vi "Acquisition Message Loop.vi"(8 "error in (no error)":errorcluster, 9 "queue out":refnum<queue>, 10 "Data Notifier":refnum<notifier>, 11 "Message Queues":T1) -> (0 "error out":errorcluster)   [LabVIEW 2022 SP3, in "Acquisition.lvlib"]
doc: "Message loop for handling messages pertaining to the acquisition of data from the hardware."
uses:
  Acquisition.lvlib
  support/Message Queue/Message Cluster.ctl
  Acquisition State.ctl
  GlobalVariable/GlobalDisconnected.vi
  GlobalVariable/GlobalFirstRep.vi
  GlobalVariable/GlobalPowerByTime.vi
  GlobalVariable/GlobalPosXbyTime.vi
  GlobalVariable/GlobalPosYbyTime.vi
  GlobalVariable/GlobalProfileByTime.vi
  GlobalVariable/Globalt0.vi
  support/Message Queue/Enqueue Message (Single).vi
  GlobalVariable/GlobalLongueurOnde.vi
  GlobalVariable/GlobalTimeStep.vi
  <vilib>/Utility/error.llb/Error Cluster From Error Code.vi
  <vilib>/ErrorRing/Error Ring.xnode
  support/Message Queue/Message Queue.lvlib
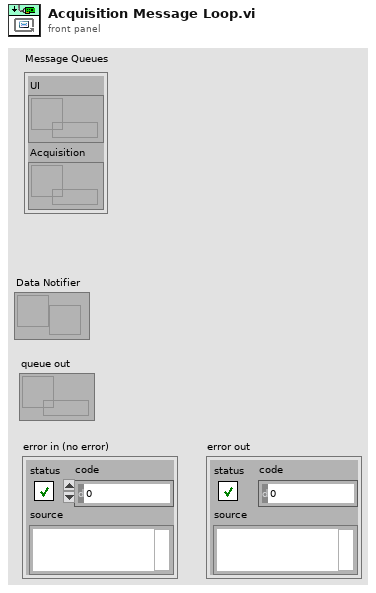
[diagram p1: front panel]
types:
  T1 = cluster{"UI":refnum<queue>, "Acquisition":refnum<queue>}
  T2 = typedef "Acquisition.lvlib/Acquisition State.ctl" = enum16{"Idle", "Acquiring"}
  T3 = enum16{"open", "replace", "create", "open or create", "replace or create", "replace or create with confirmation"}
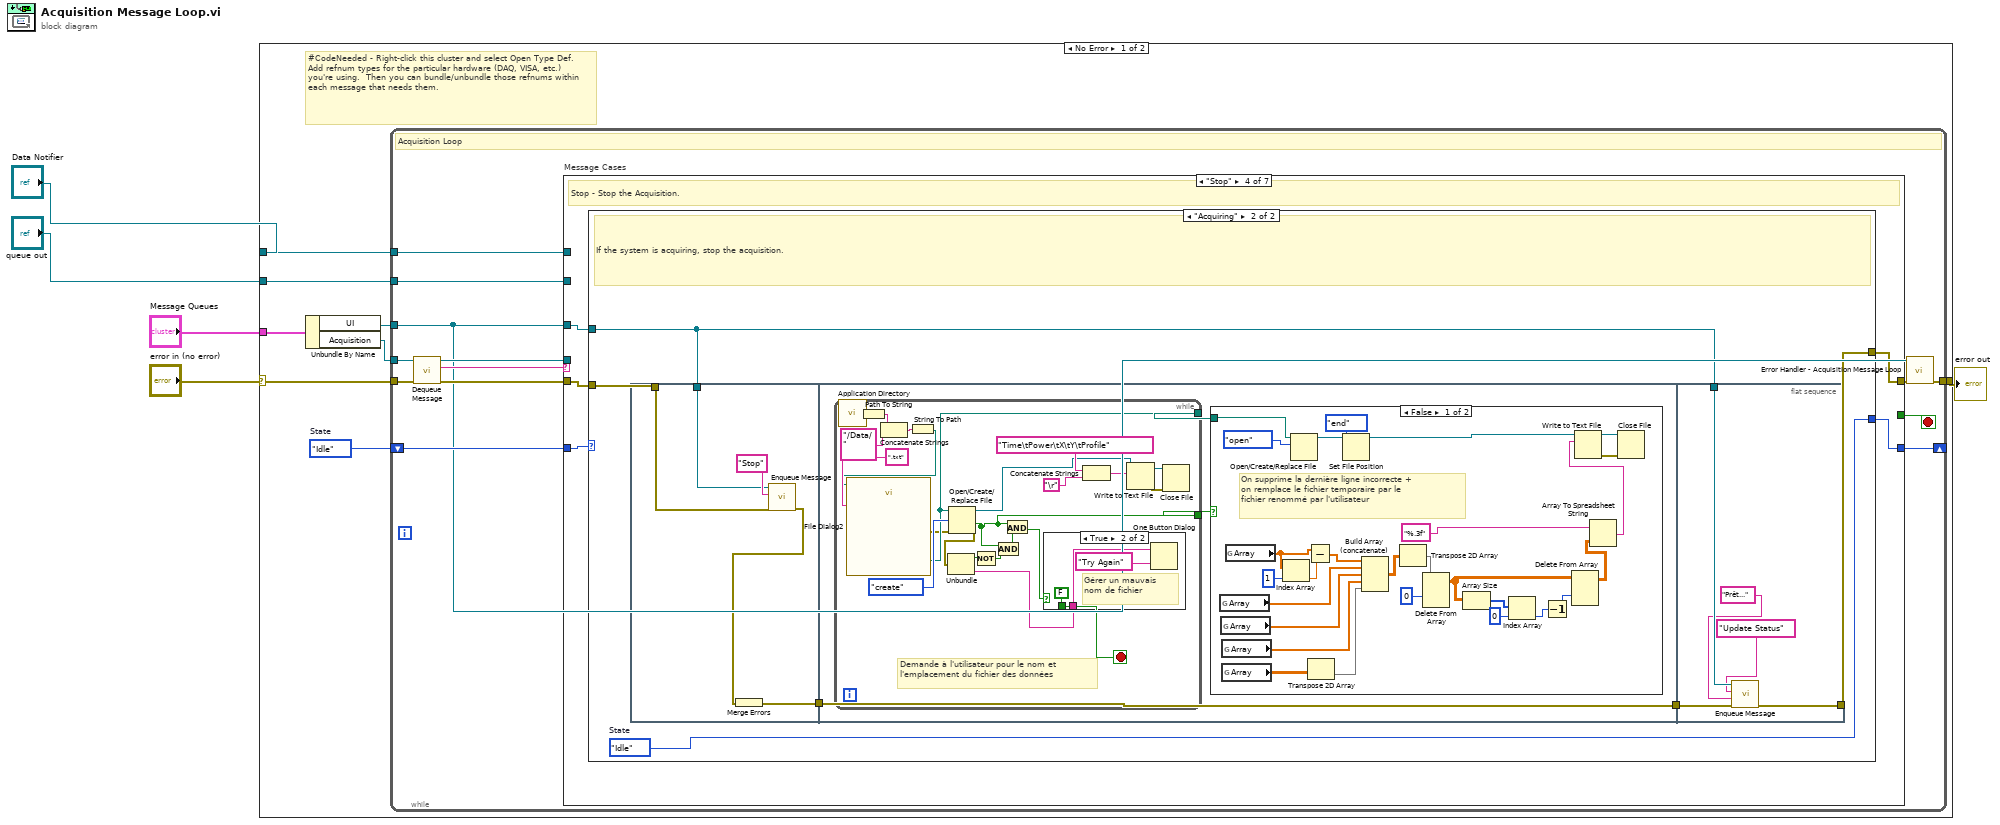
[diagram p0: block diagram]
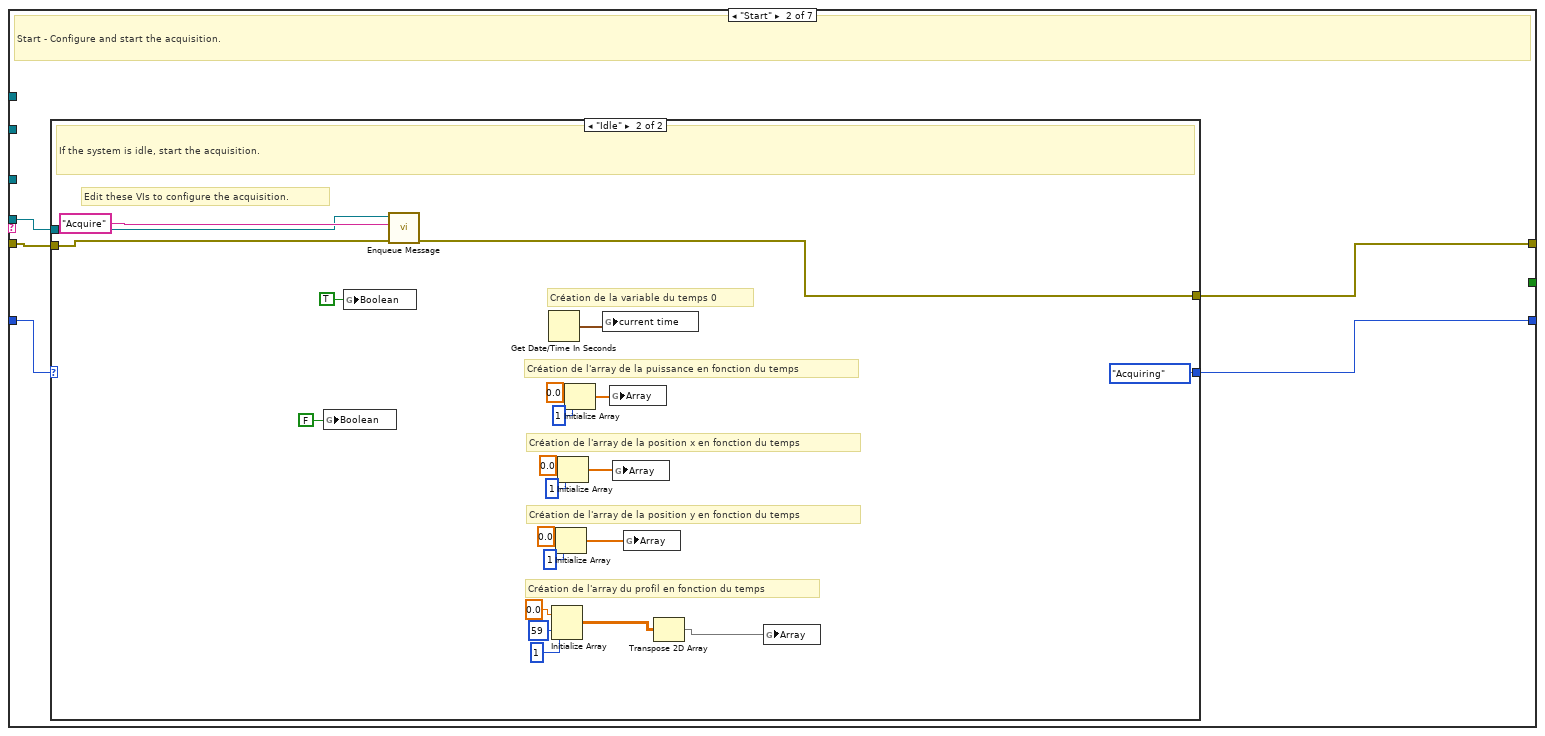
[diagram p3: hidden frame]
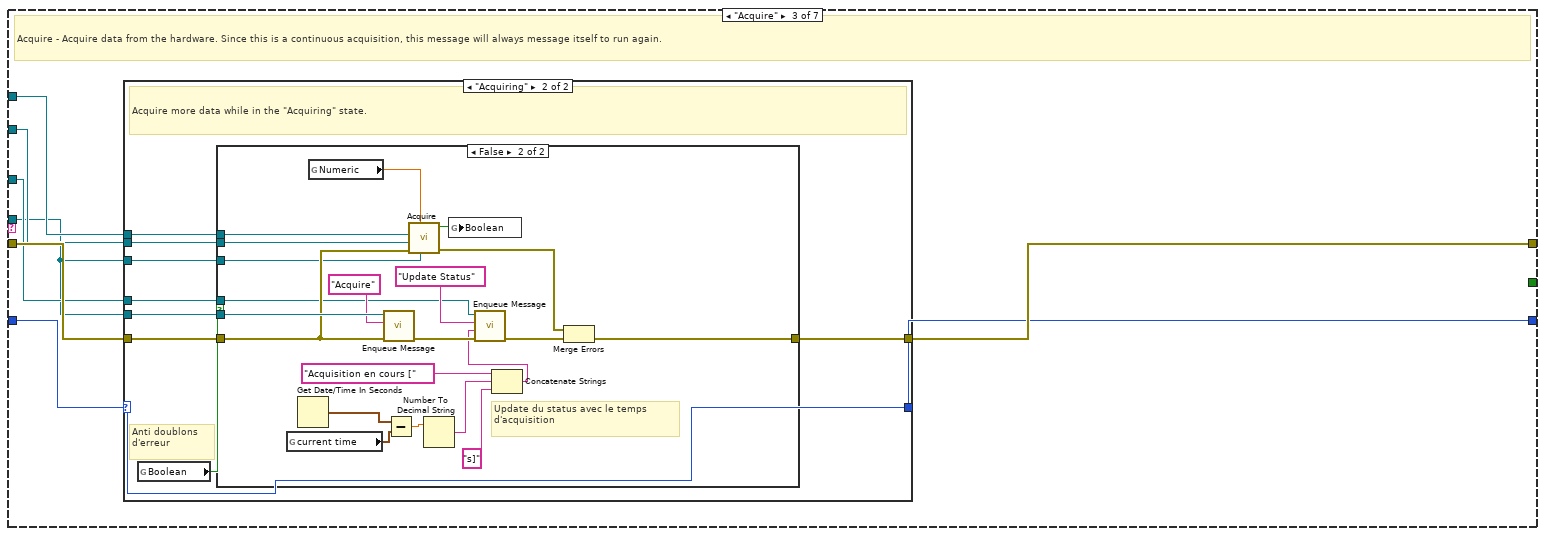
[diagram p5: hidden frame]
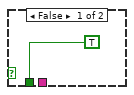
[diagram p10: hidden frame]
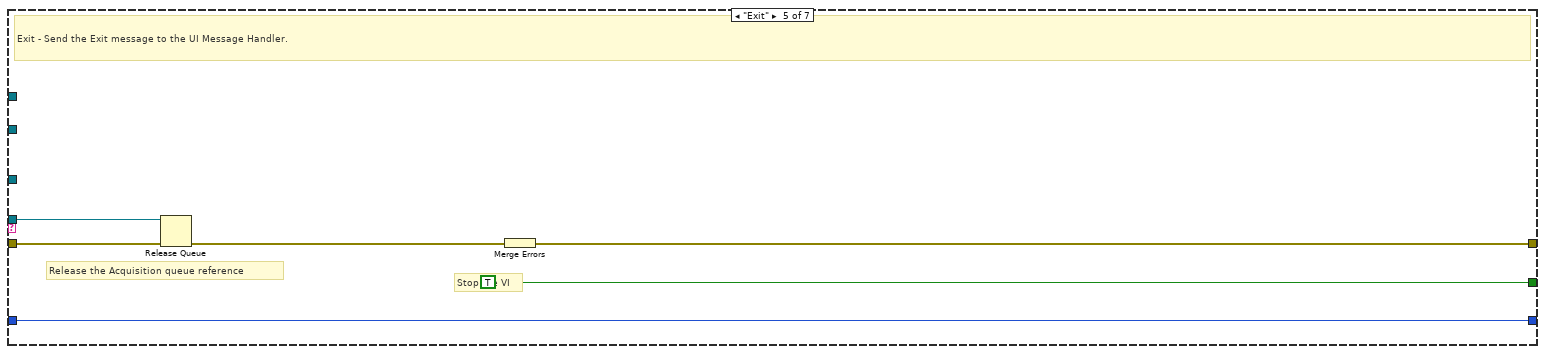
[diagram p11: hidden frame]
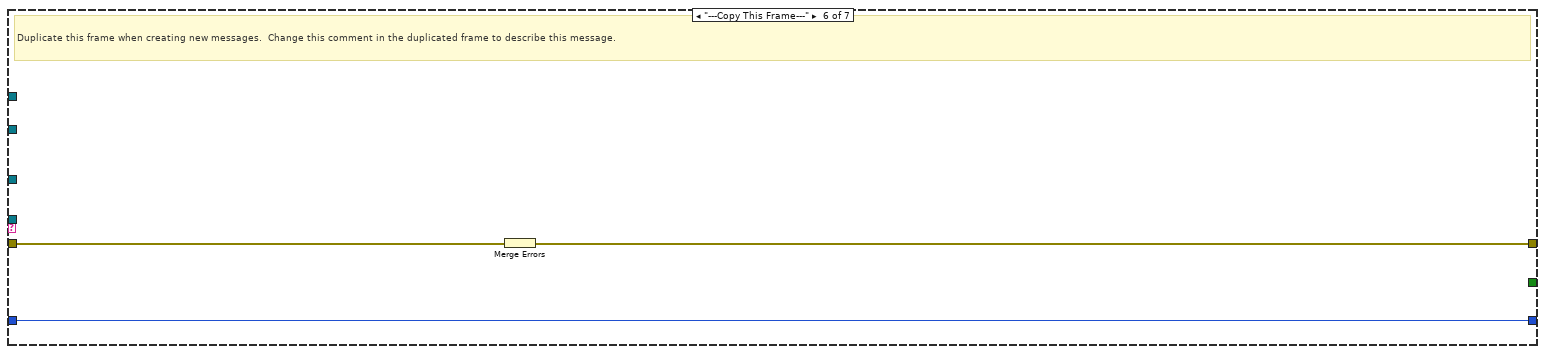
[diagram p12: hidden frame]
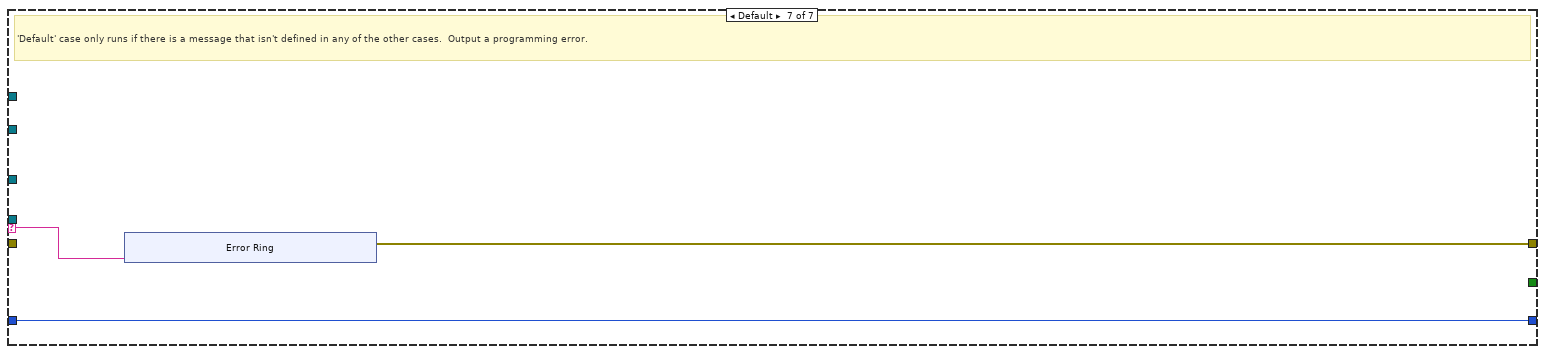
[diagram p13: hidden frame]
diagram:
  n1 = case shown="No Error" "error in (no error)" {
    selector: "error in (no error)" -> [w10 w198]
    tunnel: "Message Queues" -> [w13 _]
    tunnel: [w11 w198] -> w4
    tunnel: "Data Notifier" -> [w8 _]
    tunnel: "queue out" -> [w7 _]
    frame No Error {
      w6 = Acquisition_State."Idle"  # State
      # "#CodeNeeded - Right-click this cluster and select Open Type Def.  Add refnum types for the particular hardware (DAQ, VISA, etc.) you're using.  Then you can bundle/unbundle those refnums within each message that needs them."
      n2 = Unbundle By Name(w13) -> ("UI"=w9:refnum<queue>, "Acquisition"=w12:refnum<queue>)
      n3 = while {
        tunnel: w12 -> [w14]
        tunnel: w9 -> [w15]
        tunnel: w8 -> [w22]
        tunnel: w7 -> [w21]
        shift-right: [w19] -> _
        shift-left: w6 -> [w20]
        tunnel: w10 -> [w25]
        tunnel: [w18] -> w11
        stop <- w26 stop-if-true
        # "Acquisition Loop"
        n4 = call "Dequeue Message.vi"("error in (no error)"=w25, "Message Queue"=w14) -> ("error out"=w24:errorcluster, "Message"=w23:string, "dup Message Queue"=w16:refnum<queue>)  [unwired: 6 in, 1 out]
        n5 = case "Message Cases" shown="\"Stop\"" w23 {
          selector: w23 -> [_ _ _ _ _ _ w188]
          tunnel: w16 -> [_ w31 w58 _ w180 _ _]
          tunnel: w24 -> [w28 w32 w64 w102 w182 w187 _]
          tunnel: [w28 w33 w65 w100 w183 w186 w189] -> w17
          tunnel: [_ _ _ _ TRUE _ _] -> w26
          tunnel: w15 -> [_ _ w59 w101 _ _ _]
          tunnel: w22 -> [_ _ w63 _ _ _ _]
          tunnel: w21 -> [_ _ w62 _ _ _ _]
          tunnel: w20 -> [w27 w29 w60 w103 w179 w185 w190]
          tunnel: [w27 w30 w61 w99 w179 w185 w190] -> w19
          frame "Initialize" {
            # "Initialize  - Initialize is currently a no-op.  The hardware initialization takes place in the 'Start' message."
          }
          frame "Start" {
            # "Start - Configure and start the acquisition."
            n6 = case shown="\"Idle\"" w29 {
              selector: w29 -> [w34 _]
              tunnel: [w35 w53] -> w33
              tunnel: w32 -> [w35 w57]
              tunnel: w31 -> [_ w54]
              tunnel: [w34 Acquisition_State."Acquiring" ("Acquisition State")] -> w30
              frame "Acquiring" {
                # "The system is already acquiring. Ignore the \"Start\" message."
              }
              frame "Idle" {
                # "Création de la variable du temps 0"
                # "Création de l'array du profil en fonction du temps"
                # "Création de l'array de la position y en fonction du temps"
                # "Création de l'array de la position x en fonction du temps"
                # "Création de l'array de la puissance en fonction du temps"
                # "Edit these VIs to configure the acquisition."
                # "If the system is idle, start the acquisition."
                n7 = global write "GlobalDisconnected.vi" "Boolean"(FALSE) -> ()
                n8 = global write "GlobalFirstRep.vi" "Boolean"(TRUE ("Boolean")) -> ()
                n9 = call-poly "Enqueue Message.vi"("error in (no error)"=w57, "Message"="Acquire", "Message Queue"=w54) -> ("error out"=w53:errorcluster)  [unwired: 7 in, 1 out]
                n10 = Get Date/Time In Seconds() -> (seconds since 1Jan1904=w36:timestamp)
                n11 = Initialize Array(0.0, 59 ("dimension size"), 1 ("dimension size")) -> (w49:dbl[][])
                n12 = Initialize Array(0.0, 1) -> (w50:dbl[])
                n13 = Initialize Array(0.0, 1) -> (w51:dbl[])
                n14 = Initialize Array(0.0, 1) -> (w52:dbl[])
                n15 = global write "Globalt0.vi" "current time"(w36) -> ()
                n16 = global write "GlobalPowerByTime.vi" "Array"(w52) -> ()
                n17 = global write "GlobalPosXbyTime.vi" "Array"(w51) -> ()
                n18 = global write "GlobalPosYbyTime.vi" "Array"(w50) -> ()
                n19 = Transpose 2D Array(2D array=w49) -> (transposed array=w48:dbl[][])
                n20 = global write "GlobalProfileByTime.vi" "Array"(w48) -> ()
              }
            }
          }
          frame "Acquire" {
            # "Acquire - Acquire data from the hardware. Since this is a continuous acquisition, this message will always message itself to run again."
            n21 = case shown="\"Acquiring\"" w60 {
              selector: w60 -> [w66 w72]
              tunnel: [w67 w76] -> w65
              tunnel: w58 -> [_ w75]
              tunnel: w64 -> [w67 w71]
              tunnel: w63 -> [_ w74]
              tunnel: w62 -> [_ w73]
              tunnel: [w66 w72] -> w61
              tunnel: w59 -> [_ w70]
              tunnel: w58 -> [_ w69]
              frame "Idle" {
                # "Ignore \"Acquire\" messages when the acquisition is idle."
              }
              frame "Acquiring" {
                # "Anti doublons\nd'erreur"
                # "Acquire more data while in the \"Acquiring\" state."
                n22 = global read "GlobalDisconnected.vi" "Boolean"() -> (w68:bool)
                n23 = case shown="False" w68 {
                  tunnel: [w77 w98] -> w76
                  tunnel: w75 -> [_ w97]
                  tunnel: w74 -> [_ w94]
                  tunnel: w73 -> [_ w93]
                  tunnel: w71 -> [w77 w92]
                  tunnel: w70 -> [_ w81]
                  tunnel: w69 -> [_ w80]
                  frame True {
                  }
                  frame False {
                    # "Update du status avec le temps\nd'acquisition"
                    n24 = global read "Globalt0.vi" "current time"() -> (w87:timestamp)
                    n25 = Get Date/Time In Seconds() -> (seconds since 1Jan1904=w86:timestamp)
                    n26 = global read "GlobalLongueurOnde.vi" "Numeric"() -> (w79:dbl)
                    n27 = call-poly "Enqueue Message.vi"("error in (no error)"=w92, "Message"="Acquire", "Message Queue"=w97) -> ("error out"=w90:errorcluster)  [unwired: 7 in, 1 out]
                    n28 = Subtract(x=w86, y=w87) -> (x-y=w88:dbl)
                    n29 = call "Acquire.vi"("Acquisition"=w80, "Longueur d'onde"=w79, "error in (no error)"=w92, "Data Queue"=w93, "Data Notifier"=w94) -> ("error out"=w96:errorcluster, "Disconnected"=w78:bool)  [unwired: 5 in]
                    n30 = Number To Decimal String(number=w88) -> (decimal integer string=w85:string)  [unwired: 1 in]
                    n31 = global write "GlobalDisconnected.vi" "Boolean"(w78) -> ()
                    n32 = Concatenate Strings("Acquisition en cours [", w85, "s]" ("string")) -> (w83:string)
                    n33 = call-poly "Enqueue Message.vi"("error in (no error)"=w90, "Message Data"=w83, "Message"="Update Status", "Message Queue"=w81) -> ("error out"=w91:errorcluster)  [unwired: 6 in, 1 out]
                    n34 = Merge Errors(w96, w91) -> (w98:errorcluster)
                  }
                }
              }
            }
          }
          frame "Stop" {
            # "Stop - Stop the Acquisition."
            n35 = case shown="\"Acquiring\"" w103 {
              selector: w103 -> [w105 _]
              tunnel: w102 -> [w104 w110]
              tunnel: w101 -> [_ w106]
              tunnel: [w104 w109] -> w100
              tunnel: [w105 w108] -> w99
              frame "Idle" {
                # "The system is already idle. Ignore the \"Stop\" message."
              }
              frame "Acquiring" {
                w108 = Acquisition_State."Idle"  # State
                # "If the system is acquiring, stop the acquisition."
                n36 = flat-sequence {
                  tunnel: [w116] -> w111
                  tunnel: w106 -> [w113]
                  tunnel: w110 -> [w112]
                  tunnel: w111 -> [w118]
                  tunnel: [w118] -> w107
                  tunnel: [w177] -> w109
                  tunnel: w107 -> [w178]
                  tunnel: w106 -> [w176]
                  frame #0 {
                    n37 = call-poly "Enqueue Message.vi"("error in (no error)"=w112, "Message"="Stop", "Message Queue"=w113) -> ("error out"=w115:errorcluster)  [unwired: 7 in, 1 out]
                    n38 = Merge Errors(w115) -> (w116:errorcluster)
                  }
                  frame #1 {
                    n39 = while {
                      tunnel: [w164] -> w119
                      tunnel: [w154] -> w117
                      stop <- w160 stop-if-true
                      # "Demande à l'utilisateur pour le nom et\nl'emplacement du fichier des données"
                      n40 = call <vilib>:"Application Directory.vi"() -> ("Application Directory"=w167:path)
                      n41 = Path To String(path=w167) -> (string=w168:string)
                      n42 = Concatenate Strings(w168, "/Data/") -> (w169:string)
                      n43 = String To Path(string=w169) -> (path=w153:path)
                      n44 = call "File Dialog2"("start path"=w153, "pattern (all files)"=".txt") -> ("selected path"=w164:path, "error out"=w162:errorcluster)  [unwired: 10 in, 2 out]
                      n45 = Open/Create/Replace File(file path (use dialog)=w164, error in=w162, operation (0:open)=T3."create") -> (refnum out=w149:refnum<file>, cancelled=w154:bool, error out=w159:errorcluster)  [unwired: 3 in]
                      n46 = Unbundle(w159) -> ("status"=w158:bool, "source"=w161:string)  [unwired: 1 out]
                      n47 = Not(x=w158) -> (.not. x?=w157:bool)
                      n48 = And(x=w154, y=w157) -> (x .and. y?=w156:bool)
                      n49 = And(x=w154, y=w156) -> (x .and. y?=w155:bool)
                      n50 = case shown="True" w155 {
                        tunnel: w161 -> [_ w173]
                        tunnel: [TRUE FALSE] -> w160
                        frame False {
                        }
                        frame True {
                          # "Gérer un mauvais \nnom de fichier"
                          n51 = One Button Dialog(message=w173, button name ("OK")="Try Again") -> ()  [unwired: 1 out]
                        }
                      }
                      n52 = Concatenate Strings("Time\tPower\tX\tY\tProfile", "\r") -> (w152:string)
                      n53 = Write to Text File(file (use dialog)=w149, text=w152) -> (refnum out=w148:refnum<file>, error out=w147:errorcluster)  [unwired: 2 in, 1 out]
                      n54 = Close File(refnum=w148, error in=w147) -> ()  [unwired: 2 out]
                    }
                    n55 = case shown="False" w117 {
                      tunnel: w119 -> [w140 _]
                      frame False {
                        # "On supprime la dernière ligne incorrecte + \non remplace le fichier temporaire par le \nfichier renommé par l'utilisateur"
                        n56 = global read "GlobalPowerByTime.vi" "Array"() -> (w139:dbl[])
                        n57 = global read "GlobalPosXbyTime.vi" "Array"() -> (w138:dbl[])
                        n58 = global read "GlobalPosYbyTime.vi" "Array"() -> (w137:dbl[])
                        n59 = global read "GlobalProfileByTime.vi" "Array"() -> (w135:dbl[][])
                        n60 = global read "GlobalTimeStep.vi" "Array"() -> (w127:dbl[])
                        n61 = Index Array(array=w127, index=1) -> (element=w128:dbl)
                        n62 = Open/Create/Replace File(file path (use dialog)=w140, operation (0:open)=T3."open") -> (refnum out=w144:refnum<file>)  [unwired: 4 in, 2 out]
                        n63 = Subtract(x=w127, y=w128) -> (x-y=w126:dbl[])
                        n64 = Transpose 2D Array(2D array=w135) -> (transposed array=w134:dbl[][])
                        n65 = Set File Position(refnum=w144, from (0:start)=enum16{"start", "end", "current"}."end") -> (refnum out=w146:refnum<file>)  [unwired: 2 in, 1 out]
                        n66 = Build Array (concatenate)(w126, w139, w138, w137, w134) -> (w136:dbl[][])
                        n67 = Transpose 2D Array(2D array=w136) -> (transposed array=w130:dbl[][])
                        n68 = Delete From Array(array=w130, index (row)=0) -> (array with subset deleted=w121:dbl[][])  [unwired: 2 in, 1 out]
                        n69 = Array Size(array=w121) -> (size(s)=w125:i32[])
                        n70 = Index Array(array=w125, index=0) -> (element=w123:i32)
                        n71 = Decrement(x=w123) -> (x-1=w122:i32)
                        n72 = Delete From Array(array=w121, index (row)=w122) -> (array with subset deleted=w120:dbl[][])  [unwired: 2 in, 1 out]
                        n73 = Array To Spreadsheet String(array=w120, 3:"%.3f" ("format string")) -> (spreadsheet string=w145:string)  [unwired: 1 in]
                        n74 = Write to Text File(file (use dialog)=w146, text=w145) -> (refnum out=w133:refnum<file>, error out=w132:errorcluster)  [unwired: 2 in, 1 out]
                        n75 = Close File(refnum=w133, error in=w132) -> ()  [unwired: 2 out]
                      }
                      frame True {
                      }
                    }
                  }
                  frame #2 {
                    n76 = call-poly "Enqueue Message.vi"("error in (no error)"=w178, "Message Data"="Prêt...", "Message"="Update Status", "Message Queue"=w176) -> ("error out"=w177:errorcluster)  [unwired: 6 in, 1 out]
                  }
                }
              }
            }
          }
          frame "Exit" {
            # "Release the Acquisition queue reference"
            # "Stop the VI"
            # "Exit - Send the Exit message to the UI Message Handler."
            n77 = Release Queue(queue=w180, error in (no error)=w182) -> (error out=w181:errorcluster)  [unwired: 1 in, 2 out]
            n78 = Merge Errors(w181) -> (w183:errorcluster)
          }
          frame "---Copy This Frame---" {
            # "Duplicate this frame when creating new messages.  Change this comment in the duplicated frame to describe this message."
            n79 = Merge Errors(w187) -> (w186:errorcluster)
          }
          frame Default {
            # "'Default' case only runs if there is a message that isn't defined in any of the other cases.  Output a programming error."
            n80 = xnode "Error Ring"("parameter 0"=w188) -> ("error out"=w189:errorcluster)
          }
        }
        n81 = call "Error Handler - Acquisition Message Loop.vi"("error in (no error)"=w17, "Message Queue"=w15) -> ("dup error in"=w18:errorcluster)  [unwired: 8 in, 1 out]
      }
    }
    frame Error {
    }
  }
  "error out" <- w4
